vi "ReadDataFromClass.vi"(8 "error in (no error)":errorcluster, 11 "DataClassNotifierIn":refnum<notifier>) -> (0 "error out":errorcluster, 2 "Cluster":T1, 3 "DataClassNotifierOut":refnum<notifier>)   [LabVIEW 2013, in "Data.lvclass"]
uses:
  Data.lvclass
  DataControlType.ctl
  DataVer2.lvclass/DataVer2.lvclass
  DataVer1.lvclass/DataVer1.lvclass
  DataVer3.lvclass/DataVer3.lvclass
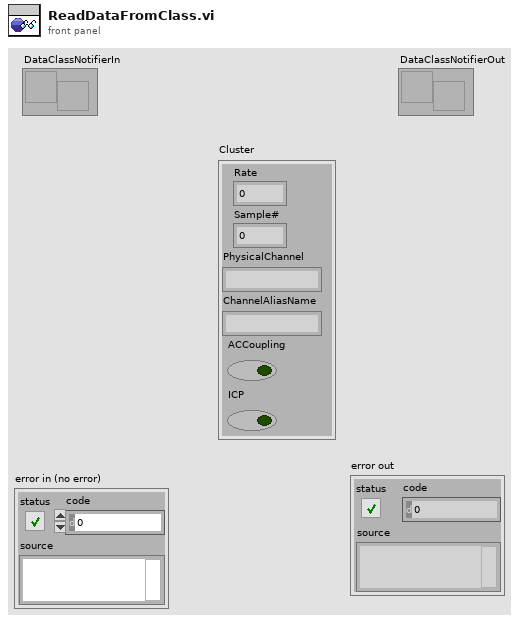
[diagram p1: front panel]
types:
  T1 = typedef "Data.lvclass/DataControlType.ctl" = cluster{"Rate":dbl, "Sample#":dbl, "PhysicalChannel":string, "ChannelAliasName":string, "ACCoupling":bool, "ICP":bool}
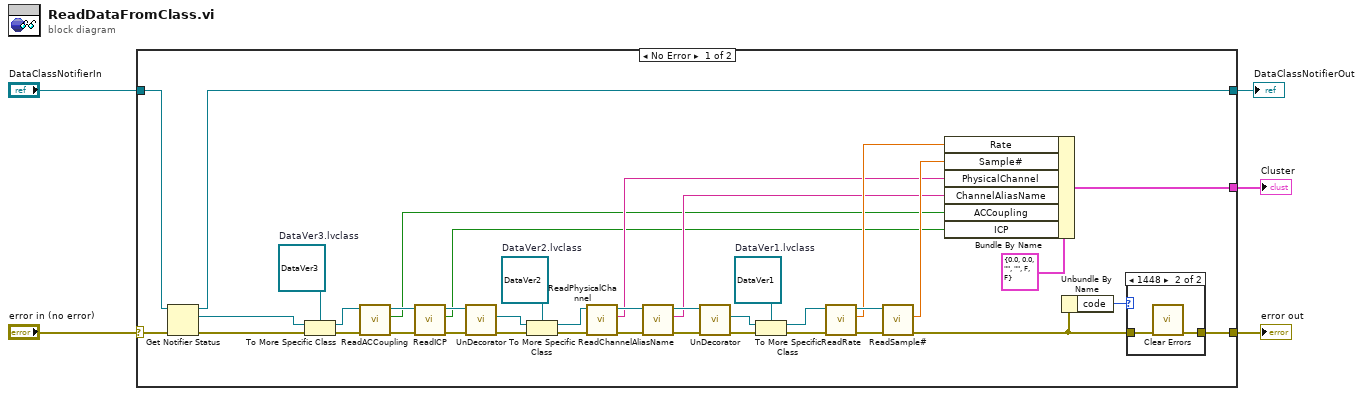
[diagram p0: block diagram]
diagram:
  n1 = case shown="No Error" "error in (no error)" {
    selector: "error in (no error)" -> [w40 w48]
    tunnel: [w6 w48] -> w5
    tunnel: [w44 _] -> w4
    tunnel: "DataClassNotifierIn" -> [w43 w49]
    tunnel: [w42 w49] -> w1
    frame No Error {
      w9 = refnum<class "DataVer3.lvclass"> refnum  # DataVer3.lvclass
      w24 = refnum<class "DataVer1.lvclass"> refnum  # DataVer1.lvclass
      w33 = refnum<class "DataVer2.lvclass"> refnum  # DataVer2.lvclass
      n2 = Get Notifier Status(notifier=w43, error in (no error)=w40) -> (notifier out=w42:refnum<notifier>, current notification=w41:refnum<class "Data.lvclass">, error out=w39:errorcluster)  [unwired: 2 out]
      n3 = To More Specific Class(target class=w9, reference=w41, error in=w39) -> (specific class reference=w10:refnum<class "DataVer3.lvclass">, error out=w11:errorcluster)
      n4 = call-dynamic "ReadACCoupling.vi"("error in (no error)"=w11, "DataVer3 in"=w10) -> ("error out"=w35:errorcluster, "ACCoupling"=w12:bool, "DataVer3 out"=w38:refnum<class "DataVer3.lvclass">)  [unwired: 7 in]
      n5 = call-dynamic "ReadICP.vi"("error in (no error)"=w35, "DataVer3 in"=w38) -> ("error out"=w36:errorcluster, "ICP"=w13:bool, "DataVer3 out"=w37:refnum<class "DataVer3.lvclass">)  [unwired: 7 in]
      n6 = call-dynamic "UnDecorator.vi"("error in (no error)"=w36, "DataVer3 in"=w37) -> ("error out"=w32:errorcluster, "DecoratorData Out"=w34:refnum<class "Data.lvclass">)  [unwired: 7 in, 1 out]
      n7 = To More Specific Class(target class=w33, reference=w34, error in=w32) -> (specific class reference=w31:refnum<class "DataVer2.lvclass">, error out=w30:errorcluster)
      n8 = call-dynamic "ReadPhysicalChannel.vi"("error in (no error)"=w30, "DataVer2 in"=w31) -> ("error out"=w28:errorcluster, "PhysicalChannel"=w15:string, "DataVer2 out"=w29:refnum<class "DataVer2.lvclass">)  [unwired: 7 in]
      n9 = call-dynamic "ReadChannelAliasName.vi"("error in (no error)"=w28, "DataVer2 in"=w29) -> ("error out"=w26:errorcluster, "ChannelAliasName"=w14:string, "DataVer2 out"=w27:refnum<class "DataVer2.lvclass">)  [unwired: 7 in]
      n10 = call-dynamic "UnDecorator.vi"("error in (no error)"=w26, "DataVer2 in"=w27) -> ("error out"=w23:errorcluster, "DecoratorData Out"=w25:refnum<class "Data.lvclass">)  [unwired: 7 in, 1 out]
      n11 = To More Specific Class(target class=w24, reference=w25, error in=w23) -> (specific class reference=w22:refnum<class "DataVer1.lvclass">, error out=w21:errorcluster)
      n12 = call-dynamic "ReadRate.vi"("error in (no error)"=w21, "DataVer1 in"=w22) -> ("error out"=w19:errorcluster, "Rate"=w17:dbl, "DataVer1 out"=w20:refnum<class "DataVer1.lvclass">)  [unwired: 7 in]
      n13 = call-dynamic "ReadSample#.vi"("error in (no error)"=w19, "DataVer1 in"=w20) -> ("error out"=w7:errorcluster, "Sample#"=w16:dbl)  [unwired: 7 in, 1 out]
      n14 = Bundle By Name(cluster=T1 {"Rate"=0.0, "Sample#"=0.0, "PhysicalChannel"="", "ChannelAliasName"="", "ACCoupling"=FALSE, "ICP"=FALSE} ("Cluster"), "Rate"=w17, "Sample#"=w16, "PhysicalChannel"=w15, "ChannelAliasName"=w14, "ACCoupling"=w12, "ICP"=w13) -> (w44:T1)
      n15 = Unbundle By Name(w7) -> ("code"=w8:i32)
      n16 = case shown="1448" w8 {
        tunnel: w7 -> [w45 w47]
        tunnel: [w45 w46] -> w6
        frame 0, Default {
        }
        frame 1448 {
          n17 = call <vilib>:"Clear Errors.vi"("error in (no error)"=w47) -> ("error out"=w46:errorcluster)  [unwired: 6 in]
        }
      }
    }
    frame Error {
    }
  }
  "Cluster" <- w4
  "error out" <- w5
  "DataClassNotifierOut" <- w1
